vi "encodeBoolean.vi"(8 "error in (no error)":errorcluster, 10 "Variant":variant) -> (0 "error out":errorcluster, 2 "Array":u8[](array[numeric]) format="%.0x")   [LabVIEW 2016, in "MsgPack.lvlib"]
uses:
  MsgPack.lvlib
  <vilib>/Utility/Data Type/NI_Data Type.lvlib
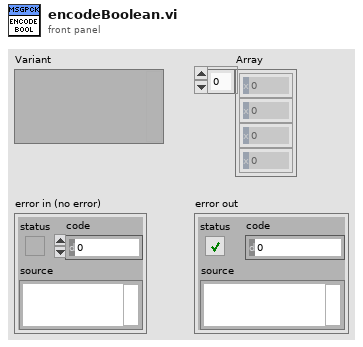
[diagram p1: front panel]
types:
  T1 = typedef "NI_Data Type.lvlib/Data Type.ctl" = enum8{"Invalid Type", "Void", "I8", "I16", "I32", "I64", "U8", "U16", "U32", "U64", "Single Float", "Double Float", "Extended Float", "Single Complex", "Double Complex", "Extended Complex", "Enum U8", "Enum U16", "Enum U32", "Enum U64", "Single Float With Unit", "Double Float With Unit", "Extended Float With Unit", "Single Complex with Unit", "Double Complex with Unit", "Extended Complex with Unit", "Boolean", "String", "Path", "Picture", "Tag", "Array", "Cluster", "Variant", "LV Variant", "Waveform", "Timestamp", "Digital Waveform", "Digital Data", "ExpressData", "Refnum", "External Data", "VI", "Poly VI", "LabVIEW Class Instance", "Fixed Point"}
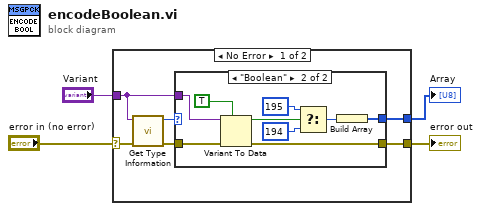
[diagram p0: block diagram]
diagram:
  n1 = case shown="No Error" "error in (no error)" {
    selector: "error in (no error)" -> [w5 w21]
    tunnel: "Variant" -> [w8 _]
    tunnel: [w7 _] -> w3
    tunnel: [w6 w21] -> w2
    frame No Error {
      n2 = call <vilib>:"Get Type Information.vi"("error in (no error)"=w5, "Variant"=w8) -> ("error out"=w9:errorcluster, "Type"=w10:T1)  [unwired: 5 in, 3 out]
      n3 = case shown="\"Boolean\"" w10 {
        tunnel: w9 -> [w11 w20]
        tunnel: w8 -> [_ w19]
        tunnel: [_ w18] -> w7
        tunnel: [w11 w14] -> w6
        frame "Invalid Type", Default {
        }
        frame "Boolean" {
          n4 = Variant To Data(error in=w20, type=TRUE, Variant=w19) -> (data=w12:bool, error out=w14:errorcluster)
          n5 = Select(t=u8 195, s=w12, f=u8 194) -> (s? t:f=w16:u8)
          n6 = Build Array(w16) -> (w18:u8[])
        }
      }
    }
    frame Error {
    }
  }
  "Array" <- w3
  "error out" <- w2
